vi "Setpwm.vi"(0 "PCA in":refnum<class "PCA.lvclass">, 5 "Led num":u8, 7 "on":u16, 9 "off":u16, 11 "error in (no error)":errorcluster) -> (4 "PCA out":refnum<class "PCA.lvclass">, 8 "OK":u8, 15 "error out":errorcluster)   [LabVIEW 2022 SP3, in "PCA9685.lvlib" / "PCA.lvclass"]
uses:
  PCA.lvclass
  PCA.lvclass/PCA.ctl
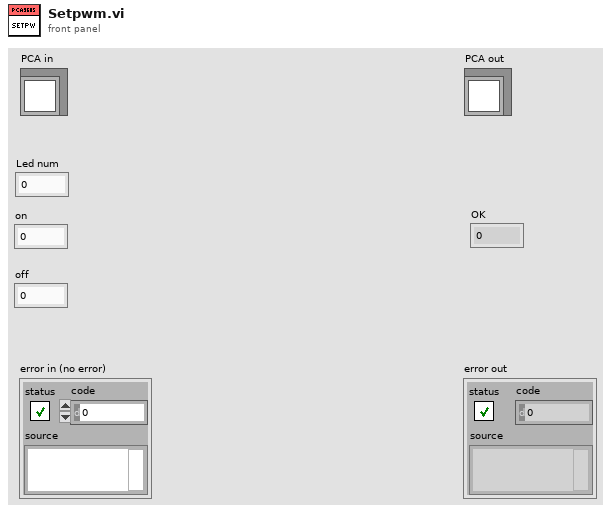
[diagram p1: front panel]
types:
  T1 = typedef "PCA9685.lvlib/PCA.lvclass/Led.ctl" = cluster{"Led_onL":i8, "Led_onH":i8, "Led_offL":i8, "Led_offH":i8}
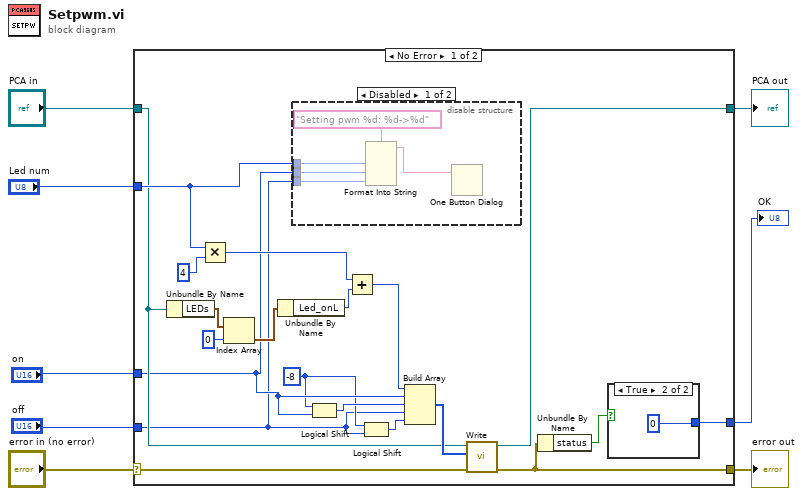
[diagram p0: block diagram]
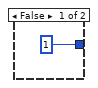
[diagram p2: hidden frame]
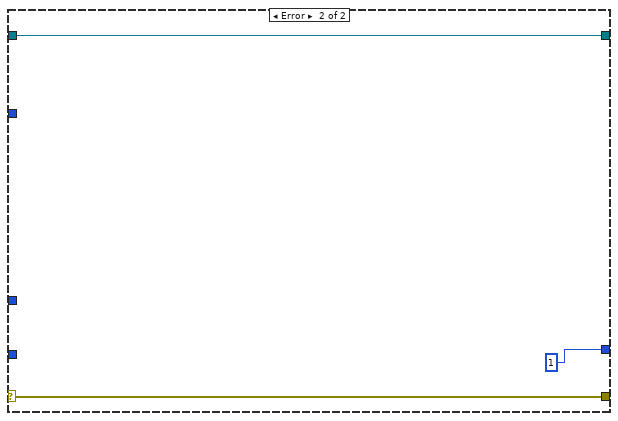
[diagram p4: hidden frame]
diagram:
  n1 = case shown="No Error" "error in (no error)" {
    selector: "error in (no error)" -> [w28 w38]
    tunnel: [w27 w38] -> w7
    tunnel: [w24 w37] -> w5
    tunnel: "PCA in" -> [w17 w37]
    tunnel: "Led num" -> [w22 _]
    tunnel: "on" -> [w12 _]
    tunnel: "off" -> [w10 _]
    tunnel: [w26 u8 1 ("Led num")] -> w1
    frame No Error {
      w11 = i16 -8 ("y")
      n2 = Unbundle By Name(w17) -> ("LEDs"=w20:T1[])
      n3 = Multiply(x=w22, y=4) -> (x*y=w15:i32)
      n4 = Index Array(array=w20, index=0) -> (element=w18:T1)
      n5 = Unbundle By Name(w18) -> ("Led_onL"=w16:i8)
      n6 = disable-structure shown="Disabled" {
        disable-tunnel: w22 -> [w34 _]
        disable-tunnel: w12 -> [w33 _]
        disable-tunnel: w10 -> [w32 _]
        frame Disabled {
          n7 = Format Into String(format string="Setting pwm %d: %d->%d", w34, w33, w32) -> (resulting string=w31:string)  [unwired: 2 in, 1 out]
          n8 = One Button Dialog(message=w31) -> ()  [unwired: 1 in, 1 out]
        }
        frame Enabled {
        }
      }
      n9 = Logical Shift(y=w11, x=w12) -> (x << y=w13:u16)
      n10 = Add(x=w15, y=w16) -> (x+y=w14:i32)
      n11 = Logical Shift(y=w11, x=w10) -> (x << y=w9:u16)
      n12 = Build Array(w14, w12, w13, w10, w9) -> (w25:i32[])
      n13 = call "Write.vi"("error in (no error)"=w28, "Data"=w25, "PCA in"=w17) -> ("error out"=w27:errorcluster, "PCA out"=w24:refnum<class "PCA.lvclass">)  [unwired: 7 in]
      n14 = Unbundle By Name(w27) -> ("status"=w23:bool)
      n15 = case shown="True" w23 {
        tunnel: [u8 1 ("Led num") 0] -> w26
        frame False {
        }
        frame True {
        }
      }
    }
    frame Error {
    }
  }
  "error out" <- w7
  "PCA out" <- w5
  "OK" <- w1
